vi "Write Current step.vi"(8 "error in (no error)":errorcluster, 10 "Current step":i32, 11 "Stepper in":refnum<class "Stepper.lvclass">) -> (0 "error out":errorcluster, 3 "Stepper out":refnum<class "Stepper.lvclass">)   [LabVIEW 2021, in "Stepper.lvclass"]
uses:
  Stepper.lvclass
  Stepper.lvclass/Stepper.ctl
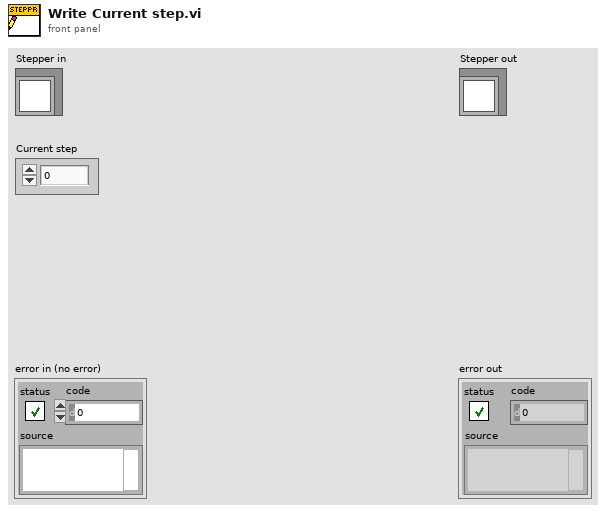
[diagram p1: front panel]
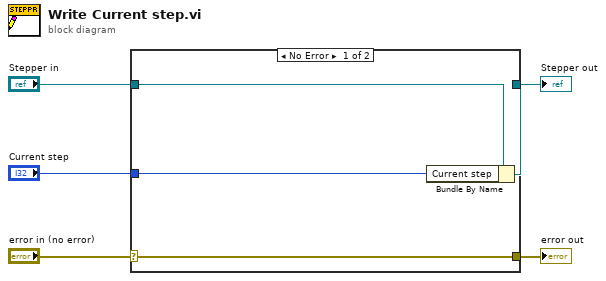
[diagram p0: block diagram]
diagram:
  n1 = case shown="No Error" "error in (no error)" {
    selector: "error in (no error)" -> [w9 w10]
    tunnel: [w9 w10] -> w4
    tunnel: [w7 w11] -> w2
    tunnel: "Stepper in" -> [w8 w11]
    tunnel: "Current step" -> [w6 _]
    frame No Error {
      n2 = Bundle By Name(cluster=w8, "Current step"=w6) -> (w7:refnum<class "Stepper.lvclass">)
    }
    frame Error {
    }
  }
  "error out" <- w4
  "Stepper out" <- w2
